vi "AIDI Test.vi"() -> ()   [LabVIEW 2015]
uses:
  AIDI/Typedefs/AIDI-Config.ctl
  AIDI/Typedefs/AIDI-Output Spec.ctl
  AIDI/Typedefs/DI-Output Spec.ctl
  AIDI/Typedefs/AIDI-Action.ctl
panel:
  out "DI Graph":dbl[][](graph)
  in  "stop":bool
  out "AI Graph":dbl[][](graph)
  in  "Config":T1={"AI"={"Channels"=["PXI1Slot4/ai0"], "Fs (Hz)"=25000.0, "Npts"=25000}, "DI"={"Channels"=[], "Fs (Hz)"=0.0, "Npts"=0, "Port"=""}, "ExtTrig"=FALSE}
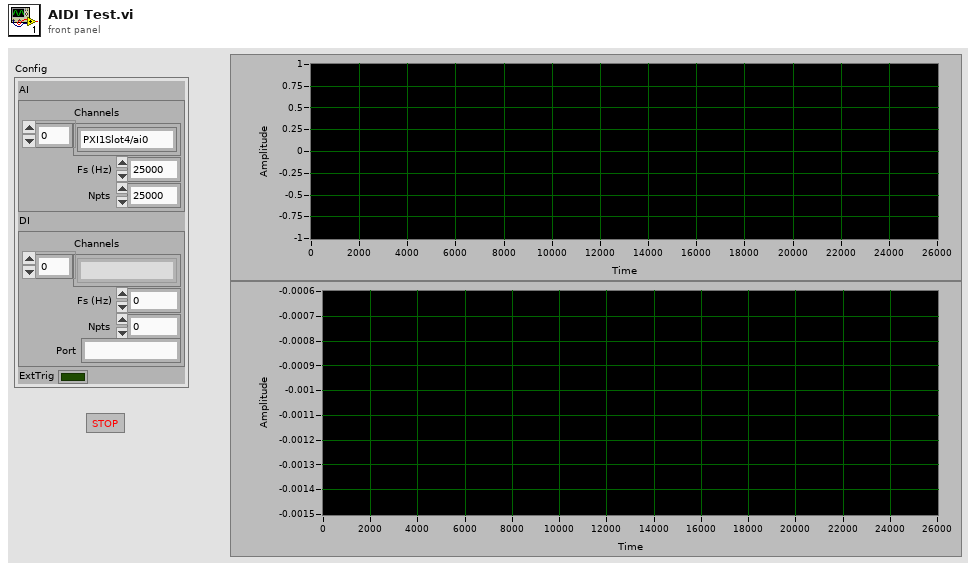
[diagram p1: front panel]
types:
  T1 = typedef "AIDI-Config.ctl" = cluster{"AI":T2, "DI":T3, "ExtTrig":bool}
  T2 = typedef "AIDI-Output Spec.ctl" = cluster{"Channels":string[], "Fs (Hz)":dbl, "Npts":i32}
  T3 = typedef "DI-Output Spec.ctl" = cluster{"Channels":string[], "Fs (Hz)":dbl, "Npts":i32, "Port":string}
  T4 = typedef "AIDI-Action.ctl" = enum16{"Configure", "Initialize", "Start", "Read", "Clean up", "Init & Start", "Config & Test", "Position"}
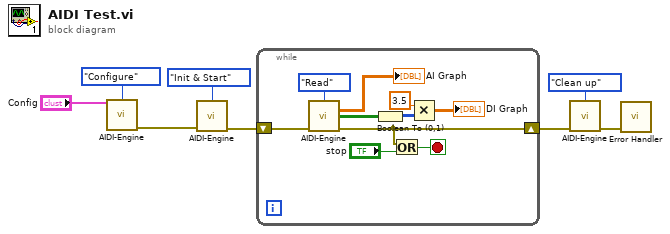
[diagram p0: block diagram]
diagram:
  n1 = call "AIDI-Engine.vi"("Config"="Config", "Action"=AIDI-Action."Configure") -> ("error out"=w2:errorcluster)  [unwired: 10 in, 3 out]
  n2 = call "AIDI-Engine.vi"("Action"=AIDI-Action."Init & Start", "error in (no error)"=w2) -> ("error out"=w7:errorcluster)  [unwired: 10 in, 3 out]
  n3 = while {
    shift-right: [w15] -> w5
    shift-left: w7 -> [w18]
    stop <- w14 stop-if-true
    n4 = call "AIDI-Engine.vi"("Action"=AIDI-Action."Read", "error in (no error)"=w18) -> ("AO"=→"AI Graph":dbl[][], "DO"=w12:bool[][], "error out"=w15:errorcluster)  [unwired: 10 in, 1 out]
    n5 = Boolean To (0,1)(Boolean=w12) -> (0, 1=w11:i16[][])
    n6 = Or(x=w15, y="stop") -> (x .or. y?=w14:bool)
    n7 = Multiply(x=3.5, y=w11) -> (x*y=→"DI Graph":dbl[][])
  }
  n8 = call "AIDI-Engine.vi"("Action"=AIDI-Action."Clean up", "error in (no error)"=w5) -> ("error out"=w4:errorcluster)  [unwired: 10 in, 3 out]
  n9 = call "Error Handler.vi"("error in (no error)"=w4) -> ()  [unwired: 13 in, 2 out]
